vi "Create Insert Shell.vi"(0 "Results":string[](array[string]), 5 "SerialNumber":string, 7 "NumberOfTesting":string, 9 "TestingStatus":string) -> (4 "Variant":variant)   [LabVIEW 2023, in "SQL Database.lvlib"]
uses:
  SQL Database.lvlib
  <vilib>/addons/database/Auxilliary.llb/DB Tools Column Info.ctl
  <vilib>/addons/database/Auxilliary.llb/DB Tools DataTypes.ctl
  <vilib>/addons/database/NI_Database_API.lvlib
panel:
  out "date/time string":string
  in  "Default database structure":T1[](array[typedef])
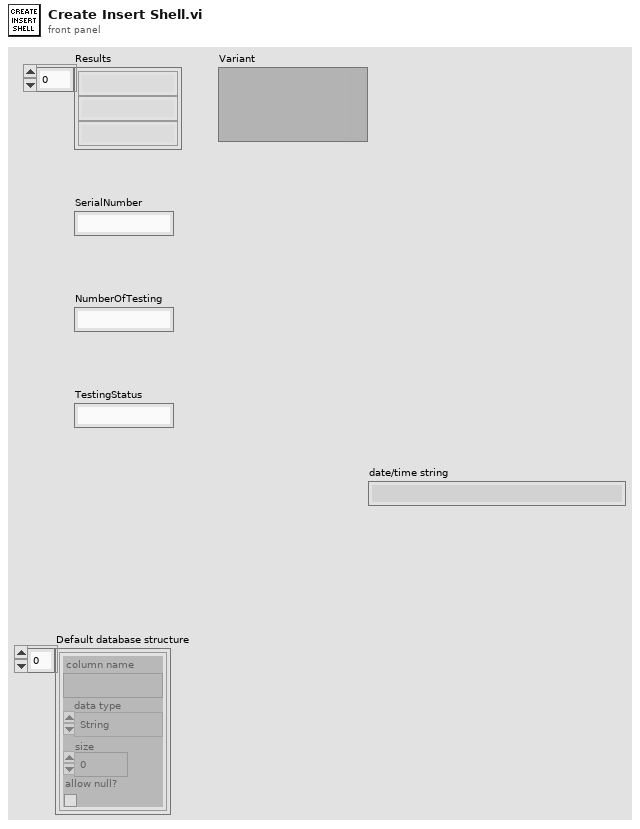
[diagram p1: front panel]
types:
  T1 = typedef "NI_Database_API.lvlib/DB Tools Column Info.ctl" = cluster{"column name":string, "data type":T2, "size":i32, "allow null?":bool}
  T2 = typedef "NI_Database_API.lvlib/DB Tools DataTypes.ctl" = enum16{"String", "Long (I32)", "Single (SGL)", "Double (DBL)", "Date/Time", "Binary"}
  T3 = cluster{"[0]":string, "[1]":string, "[2]":string, "[3]":string, "[4]":string, "[5]":string, "[6]":string, "[7]":string, "[8]":string}
  T4 = cluster{"[0]":string, "[1]":string, "[2]":string, "[3]":string, "[4]":string, "[5]":string, "[6]":string, "[7]":string, "[8]":string, "[9]":string, "[10]":string, "[11]":string, "[12]":string, "[13]":string, "[14]":string, "[15]":string, "[16]":string, "[17]":string, "[18]":string, "[19]":string, "[20]":string, "[21]":string, "[22]":string, "[23]":string, "[24]":string, "[25]":string, "[26]":string, "[27]":string, "[28]":string, "[29]":string, "[30]":string, "[31]":string, "[32]":string, "[33]":string, "[34]":string, "[35]":string, "[36]":string, "[37]":string, "[38]":string, "[39]":string, "[40]":string, "[41]":string, "[42]":string, "[43]":string, "[44]":string, "[45]":string, "[46]":string, "[47]":string, "[48]":string, "[49]":string, "[50]":string, "[51]":string, "[52]":string, "[53]":string}
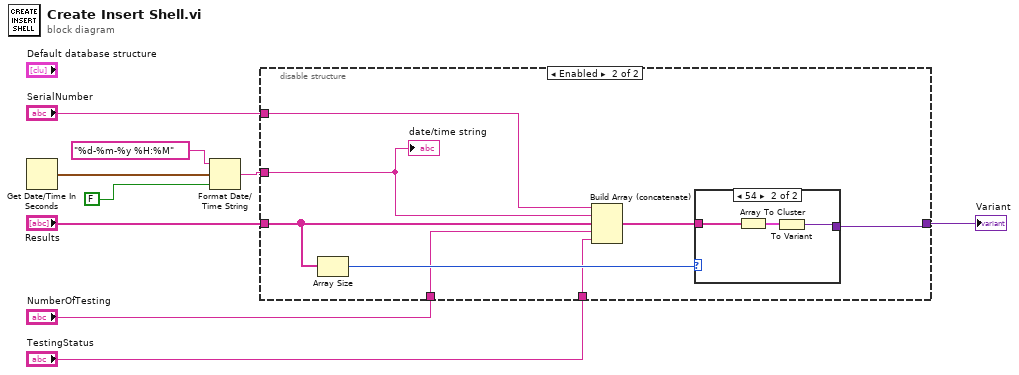
[diagram p0: block diagram]
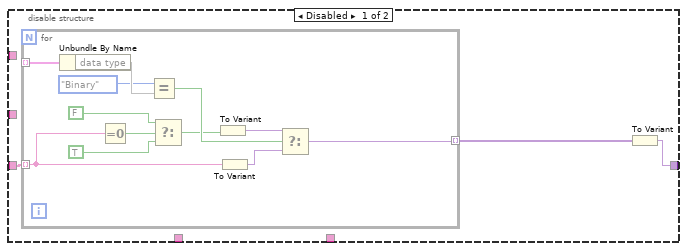
[diagram p2: hidden frame]
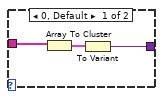
[diagram p3: hidden frame]
diagram:
  n1 = Get Date/Time In Seconds() -> (seconds since 1Jan1904=w7:timestamp)
  n2 = Format Date/Time String(time format string (%c)="%d-%m-%y %H:%M", seconds (now)=w7, UTC format=FALSE) -> (date/time string=w6:string)
  n3 = disable-structure shown="Enabled" {
    disable-tunnel: [w11 w32] -> w9
    disable-tunnel: "Results" -> [w10 w29]
    disable-tunnel: w6 -> [_ w30]
    disable-tunnel: "SerialNumber" -> [_ w31]
    disable-tunnel: "TestingStatus" -> [_ w27]
    disable-tunnel: "NumberOfTesting" -> [_ w26]
    frame Disabled {
      n4 = for {
        tunnel: [w25] -> w13 mode=indexing
        tunnel: w10 -> [w16] mode=indexing
        tunnel: [w14] -> w12 mode=indexing
        n5 = Unbundle By Name(w25) -> ("data type"=w24)
        n6 = Equal To 0?(x=w16) -> (x = 0?=w21:bool)
        n7 = Equal?(x=DB_Tools_DataTypes."Binary" ("y"), y=w24) -> (x = y?=w22:bool)
        n8 = Select(t=FALSE, s=w21, f=TRUE) -> (s? t:f=w18:bool)
        n9 = To Variant(anything=w18) -> (Variant=w17:variant)
        n10 = To Variant(anything=w16) -> (Variant=w15:variant)
        n11 = Select(t=w17, s=w22, f=w15) -> (s? t:f=w14:variant)
      }
      n12 = To Variant(anything=w12) -> (Variant=w11:variant)
    }
    frame Enabled {
      n13 = Array Size(array=w29) -> (size(s)=w33:i32)
      n14 = Build Array (concatenate)(w31, w30, w29, w26, w27) -> (w28:string[])
      n15 = case shown="54" w33 {
        tunnel: w28 -> [w36 w39]
        tunnel: [w34 w37] -> w32
        frame 0, Default {
          n16 = Array To Cluster(array=w36) -> (cluster=w35:T3)
          n17 = To Variant(anything=w35) -> (Variant=w34:variant)
        }
        frame 54 {
          n18 = Array To Cluster(array=w39) -> (cluster=w38:T4)
          n19 = To Variant(anything=w38) -> (Variant=w37:variant)
        }
      }
      "date/time string" <- w30
    }
  }
  "Variant" <- w9
